vi "nominal run number.vi"(8 "error in (no error)":errorcluster, 10 "out_number":u32, 11 "run":i32) -> (0 "error out":errorcluster, 2 "out_number out":u32, 3 "function return":i32)   [LabVIEW 2020, in "client.lvlib"]
doc: "int32_t nominal_run_number(int32_t run, uint32_t *out_number);"
uses:
  client.lvlib
  nominalClient_64.dll
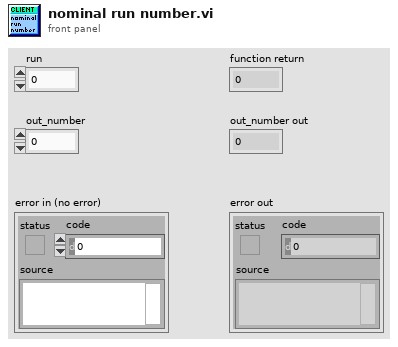
[diagram p1: front panel]
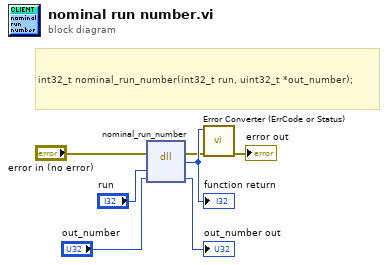
[diagram p0: block diagram]
diagram:
  # "int32_t nominal_run_number(int32_t run, uint32_t *out_number);"
  n1 = dll-call lib="C:/code/labview-client-rs/lv_src/client/nominalClient_64.*" fn="nominal_run_number"(error in="error in (no error)", "run"="run", "out_number"="out_number") -> (error out=w2:errorcluster, w7:i32, "out_number"=→"out_number out":u32)  [unwired: 3 in, 1 out]
  "function return" <- w7
  n2 = call "Error Converter (ErrCode or Status).vi"("error in (no error)"=w2, "error code"=w7) -> ("error out"=→"error out":errorcluster)  [unwired: 9 in]
